vi "Predet_Sensor_Read.vi"(8 "Error In":errorcluster, 9 "Temperature Freq":dbl, 10 "Pressure Freq":dbl, 11 "Sampling Time":dbl=1.0) -> (0 "Error Out":errorcluster, 1 "Temperature Data":waveform(dbl)[](array[waveform]), 2 "Pressure Data":waveform(dbl)[](array[waveform]))   [LabVIEW 2016]
uses:
  <vilib>/DAQmx/read.llb/DAQmx Read (Analog 1D Wfm NChan NSamp).vi
  <vilib>/DAQmx/create/channels.llb/DAQmx Create Channel (AI-Temperature-Thermocouple).vi
  <resource>/objmgr/daqmx.rc
  <vilib>/DAQmx/configure/timing.llb/DAQmx Timing (Sample Clock).vi
  <vilib>/DAQmx/create/channels.llb/DAQmx Create Channel (AI-Current-Basic).vi
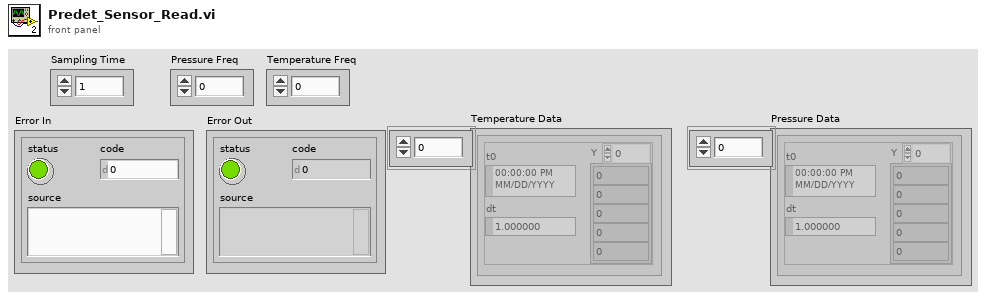
[diagram p1: front panel]
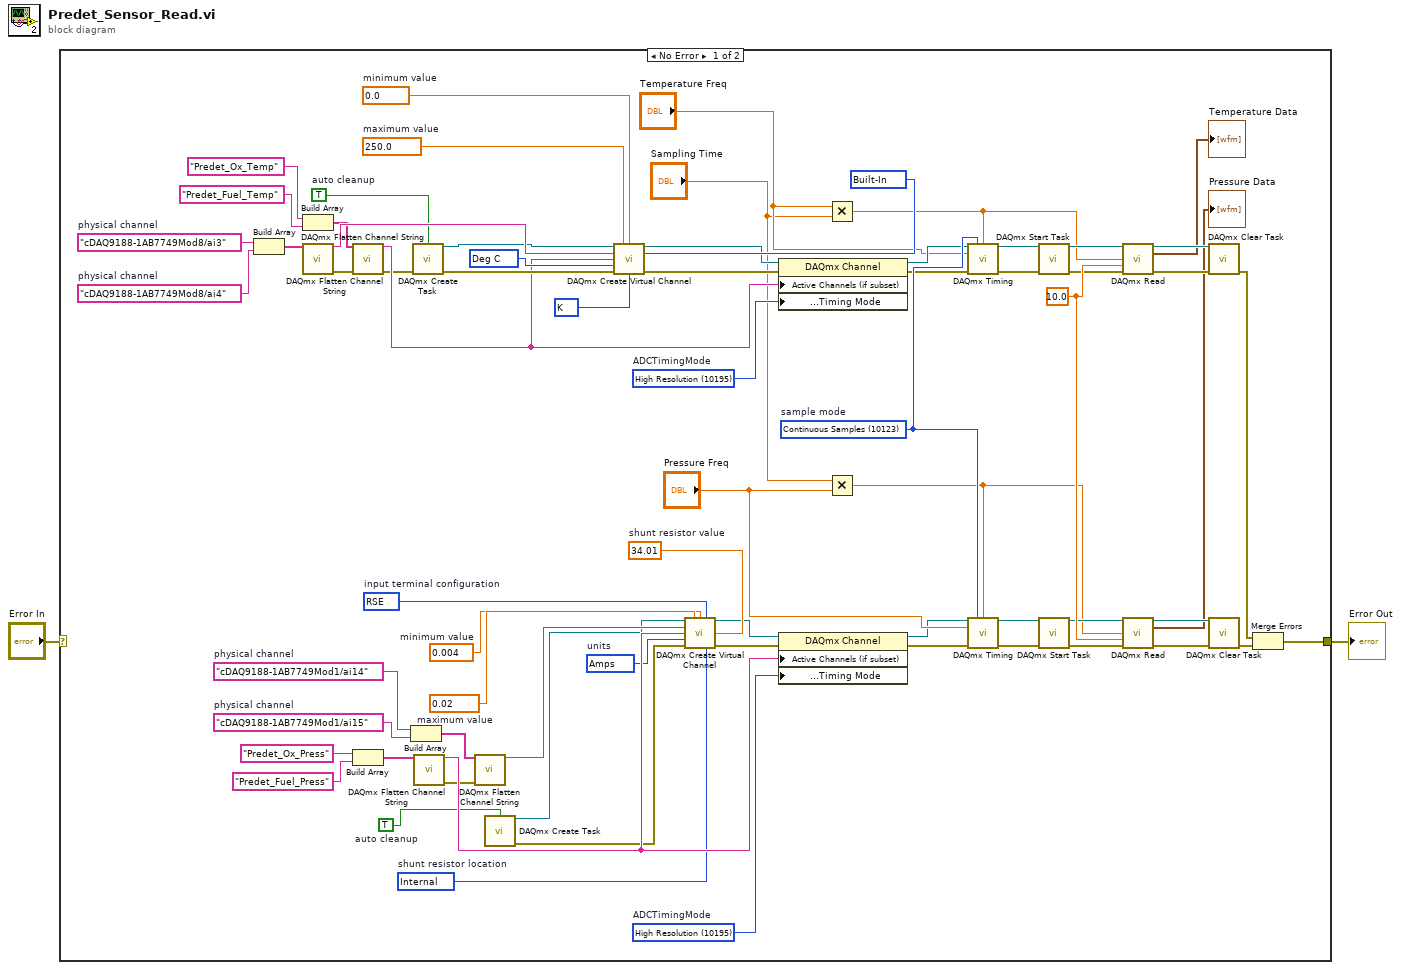
[diagram p0: block diagram]
diagram:
  n1 = case shown="No Error" "Error In" {
    selector: "Error In" -> [_ w73]
    tunnel: [w3 w73] -> w1
    frame No Error {
      w72 = 10.0 ("timeout")
      w67 = "cDAQ9188-1AB7749Mod1/ai15"  # physical channel
      w66 = "cDAQ9188-1AB7749Mod1/ai14"  # physical channel
      w71 = 10123 items=["Finite Samples"=10178, "Continuous Samples"=10123, "Hardware Timed Single Point"=12522]  # sample mode
      w50 = 10195 items=["High Resolution"=10195, "High Speed"=14712, "Best 50 Hz Rejection"=14713, "Best 60 Hz Rejection"=14714]  # ADCTimingMode
      w51 = 10083 items=["default"=-1, "RSE"=10083, "NRSE"=10078, "Differential"=10106, "Pseudodifferential"=12529]  # input terminal configuration
      w52 = 10342 items=["Amps"=10342, "From Custom Scale"=10065]  # units
      w53 = 34.01  # shunt resistor value
      w54 = 10200 items=["Internal"=10200, "External"=10167]  # shunt resistor location
      w56 = 0.004  # minimum value
      w57 = 0.02  # maximum value
      w59 = TRUE  # auto cleanup
      w45 = "cDAQ9188-1AB7749Mod8/ai4"  # physical channel
      w44 = "cDAQ9188-1AB7749Mod8/ai3"  # physical channel
      w43 = 10143 items=["Deg C"=10143, "Deg F"=10144, "Kelvins"=10325, "Deg R"=10145, "From Custom Scale"=10065] ("units")
      w42 = 10073 items=["J"=10072, "K"=10073, "N"=10077, "R"=10082, "S"=10085, "T"=10086, "B"=10047, "E"=10055] ("thermocouple type")
      w41 = 10200 items=["Built-In"=10200, "Constant Value"=10116, "Channel"=10113] ("cjc source")
      w32 = 10195 items=["High Resolution"=10195, "High Speed"=14712, "Best 50 Hz Rejection"=14713, "Best 60 Hz Rejection"=14714]  # ADCTimingMode
      w35 = 0.0  # minimum value
      w36 = 250.0  # maximum value
      w38 = TRUE  # auto cleanup
      n2 = Build Array(w44, w45) -> (w46:string[])
      n3 = Build Array("Predet_Ox_Temp" ("name to assign"), "Predet_Fuel_Temp" ("name to assign")) -> (w19:string[])
      n4 = call <vilib>:"DAQmx Flatten Channel String.vi"("names in"=w46) -> ("names out"=w40:string, "error out"=w6:errorcluster)  [unwired: 13 in]
      n5 = call <vilib>:"DAQmx Flatten Channel String.vi"("names in"=w19, "error in"=w6) -> ("names out"=w18:string, "error out"=w17:errorcluster)  [unwired: 12 in]
      n6 = Build Array("Predet_Ox_Press" ("name to assign"), "Predet_Fuel_Press" ("name to assign")) -> (w62:string[])
      n7 = Build Array(w66, w67) -> (w68:string[])
      n8 = call <vilib>:"DAQmx Create Task.vi"("auto cleanup"=w38, "error in"=w17) -> ("task out"=w37:refnum<k21>, "error out"=w39:errorcluster)  [unwired: 3 in, 9 out]
      n9 = call <vilib>:"DAQmx Flatten Channel String.vi"("names in"=w62) -> ("names out"=w63:string, "error out"=w7:errorcluster)  [unwired: 13 in]
      n10 = call <vilib>:"DAQmx Flatten Channel String.vi"("names in"=w68, "error in"=w7) -> ("names out"=w61:string)  [unwired: 12 in, 1 out]
      n11 = call <vilib>:"DAQmx Create Task.vi"("auto cleanup"=w59) -> ("task out"=w58:refnum<k21>, "error out"=w60:errorcluster)  [unwired: 4 in, 9 out]
      n12 = call-poly <vilib>:"DAQmx Create Virtual Channel.vi"("task in"=w37, "maximum value"=w36, "minimum value"=w35, "physical channels"=w40, "cjc source"=w41, "name to assign"=w18, "units"=w43, "error in"=w39, "thermocouple type"=w42) -> ("task out"=w31:refnum<k21>, "error out"=w34:errorcluster)  [unwired: 5 in]
      n13 = call-poly <vilib>:"DAQmx Create Virtual Channel.vi"("task in"=w58, "maximum value"=w57, "minimum value"=w56, "input terminal configuration"=w51, "physical channels"=w61, "name to assign"=w63, "external shunt resistor value"=w53, "units"=w52, "error in"=w60, "shunt resistor location"=w54) -> ("task out"=w49:refnum<k21>, "error out"=w55:errorcluster)  [unwired: 1 in, 3 out]
      n14 = property class="DAQmx Channel"(reference=w31, error in=w34, "Active Channels (if subset)"=w18, "Analog Input:General Properties:Digitizer/ADC:Timing Mode"=w32) -> (reference out=w30:refnum<k21>, error out=w33:errorcluster)
      n15 = property class="DAQmx Channel"(reference=w49, error in=w55, "Active Channels (if subset)"=w63, "Analog Input:General Properties:Digitizer/ADC:Timing Mode"=w50) -> (reference out=w5:refnum<k21>, error out=w4:errorcluster)
      n16 = Multiply(x="Temperature Freq", y="Sampling Time") -> (x*y=w10:dbl)
      n17 = Multiply(x="Sampling Time", y="Pressure Freq") -> (x*y=w9:dbl)
      n18 = call-poly <vilib>:"DAQmx Timing.vi"("task/channels in"=w30, "sample mode"=w71, "samples per channel"=w10, "rate"="Temperature Freq", "error in"=w33) -> ("task out"=w47:refnum<k21>, "error out"=w48:errorcluster)  [unwired: 2 in, 7 out]
      n19 = call-poly <vilib>:"DAQmx Timing.vi"("task/channels in"=w5, "sample mode"=w71, "samples per channel"=w9, "rate"="Pressure Freq", "error in"=w4) -> ("task out"=w70:refnum<k21>, "error out"=w69:errorcluster)  [unwired: 2 in, 7 out]
      n20 = call <vilib>:"DAQmx Start Task.vi"("task/channels in"=w47, "error in"=w48) -> ("task out"=w26:refnum<k21>, "error out"=w27:errorcluster)  [unwired: 12 out]
      n21 = call <vilib>:"DAQmx Start Task.vi"("task/channels in"=w70, "error in"=w69) -> ("task out"=w22:refnum<k21>, "error out"=w23:errorcluster)  [unwired: 12 out]
      n22 = call-poly <vilib>:"DAQmx Read.vi"("task/channels in"=w26, "number of samples per channel"=w10, "timeout"=w72, "error in"=w27) -> ("task out"=w29:refnum<k21>, "data"=→"Temperature Data":waveform(dbl)[], "error out"=w28:errorcluster)  [unwired: 9 out]
      n23 = call-poly <vilib>:"DAQmx Read.vi"("task/channels in"=w22, "number of samples per channel"=w9, "timeout"=w72, "error in"=w23) -> ("task out"=w25:refnum<k21>, "data"=→"Pressure Data":waveform(dbl)[], "error out"=w24:errorcluster)  [unwired: 9 out]
      n24 = call <vilib>:"DAQmx Clear Task.vi"("task in"=w29, "error in"=w28) -> ("error out"=w13:errorcluster)  [unwired: 13 out]
      n25 = call <vilib>:"DAQmx Clear Task.vi"("task in"=w25, "error in"=w24) -> ("error out"=w14:errorcluster)  [unwired: 13 out]
      n26 = Merge Errors(w13, w14) -> (w3:errorcluster)
    }
    frame Error {
    }
  }
  "Error Out" <- w1
